vi "OBDservice03.vi"(8 "错误输入（无错误）":errorcluster, 11 "diag ref out输入":T1 {"Diagostic Globals"."Fill Byte" format="%x"; "TesterPresent Message" format="%.0x"; "Selected I/O Mode" items=["CAN", "CAN FD", "CAN FD+BRS", "ECU Determined"]; "DoIP Protocol Version" items=["2010"=1, "2012"=2]; "RX_DL" items=["8"=8, "12"=12, "16"=16, "20"=20, "24"=24, "32"=32, "48"=48, "64"=64]; "TX_DL" items=["8"=8, "12"=12, "16"=16, "20"=20, "24"=24, "32"=32, "48"=48, "64"=64]; "I/O Mode" items=["CAN", "CAN FD", "CAN FD+BRS", "Not yet determined"]}) -> (0 "错误输出":errorcluster, 1 "success?":bool, 2 "dtcs":string[](array[string]), 3 "diag ref out输出":T1 {"Diagostic Globals"."Fill Byte" format="%x"; "TesterPresent Message" format="%.0x"; "Selected I/O Mode" items=["CAN", "CAN FD", "CAN FD+BRS", "ECU Determined"]; "DoIP Protocol Version" items=["2010"=1, "2012"=2]; "RX_DL" items=["8"=8, "12"=12, "16"=16, "20"=20, "24"=24, "32"=32, "48"=48, "64"=64]; "TX_DL" items=["8"=8, "12"=12, "16"=16, "20"=20, "24"=24, "32"=32, "48"=48, "64"=64]; "I/O Mode" items=["CAN", "CAN FD", "CAN FD+BRS", "Not yet determined"]})   [LabVIEW 2018]
uses:
  <vilib>/Automotive Diagnostic Command Set/Diagnostic Transport.llb/Diag Reference.ctl
  <vilib>/Automotive Diagnostic Command Set/Diagnostic Transport.llb/Transport Protocol Selector.ctl
  <vilib>/Automotive Diagnostic Command Set/Diagnostic Transport.llb/DoIP Protocol Version.ctl
  <vilib>/Automotive Diagnostic Command Set/Diagnostic Transport.llb/Diag Globals.ctl
  <vilib>/addons/Automotive Diagnostic Command Set/NI_Automotive Diagnostic Command Set.lvlib
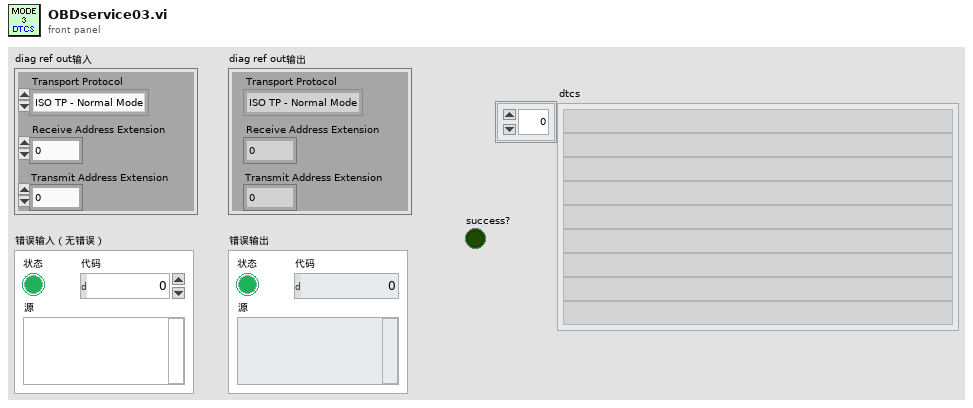
[diagram p1: front panel]
types:
  T1 = typedef "NI_Automotive Diagnostic Command Set.lvlib/Diag Reference.ctl" = cluster{"Diag CAN Handle":u32, "Transport Protocol":T2, "Receive Address Extension":u8, "Transmit Address Extension":u8, "Receive CAN Id":u32, "Transmit CAN Id":u32, "Log Frames ?":bool, "My TP Address":u8, "Other TP Address":u8, "T1":u16, "T2":u16, "T3":u16, "T4":u16, "Tx SN":u8, "Block Size":u8, "Rx SN":u8, "VW TP Initialized?":bool, "Tx block no":u8, "baud rate":u64, "Interface":string, "Channel Diag CAN Handle":u32, "UDP Connection ID":refnum<k16>, "TCP Connection ID":refnum<k5>, "Target IP Addr":u32, "Source Address":u16, "Target Address":u16, "Send Header NACK?":bool, "DLL Handle":u32, "NAD":u8, "Time Stamp read first":dbl, "Time Stamp read last":dbl, "Time Stamp write first":dbl, "Time Stamp write last":dbl, "Time Stamp write":dbl, "Time Stamp read":dbl, " I/O Mode":u32, "FD Baudrate":u64, "TX_DL":u16, "RX_DL":u16, "DoIP Protocol Version":T3, " Selected I/O Mode":u32, "TesterPresent Counter":u32, "TesterPresent Limit":u32, "TesterPresent Tick[ms]":i32, "TesterPresent RequireResponse?":bool, "TesterPresent Stored Ref?":bool, "TesterPresent Message":u8[], "TesterPresent Task Handle":i32, "TesterPresent Semaphore":T4, "Response Plausibility Check":u32, "Default Version?":bool, "Diagostic Globals":T5, "Session-based Properties?":bool}
  T2 = typedef "NI_Automotive Diagnostic Command Set.lvlib/Transport Protocol Selector.ctl" = enum16{"ISO TP - Normal Mode", "ISO TP - Mixed Mode", "VW TP 2.0", "Diagnostics on IP", "ISO TP LIN"}
  T3 = typedef "NI_Automotive Diagnostic Command Set.lvlib/DoIP Protocol Version.ctl" = u8
  T4 = typedef "Semaphore RefNum" = refnum<k1>
  T5 = typedef "NI_Automotive Diagnostic Command Set.lvlib/Diag Globals.ctl" = cluster{"Timeout FC (Bs)":u32, "Timeout CF (Cr)":u32, "Timeout Diag Command":u32, "Receive Block Size (BS)":u8, "Wait Time CF (STmin)":u8, "Max Waits (N_WFTmax)":u8, "Waits to Send (N_WAIT)":i32, "Time between Waits (TW)":u32, "Fill CAN Frames?":bool, "Fill Byte":u32, "Invalid Response as Error?":bool, "Max RspPending Count":u32, "VWTP Command Timeout":u32, "Transport Protocol":T2, "Diag CAN Handle":u32, "DLL Handle":u32, "Timeout RspPending":u32}
  T6 = typedef "Diagnostic Trouble Code.ctl" = cluster{"DTC":u32, "Status":u32, "Add Data":u32}
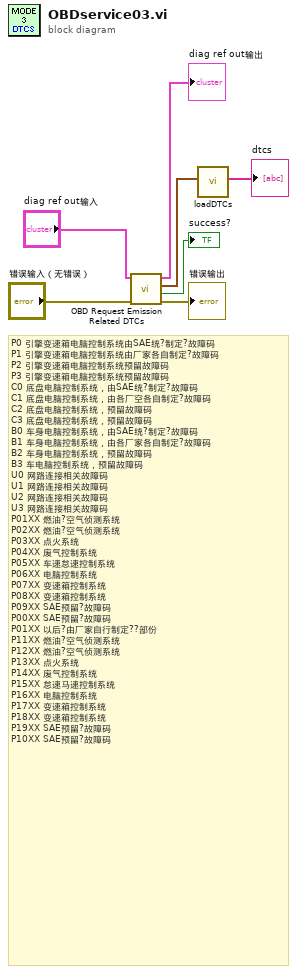
[diagram p0: block diagram]
diagram:
  # "P0 引擎变速箱电脑控制系统由SAE统?制定?故障码\nP1 引擎变速箱电脑控制系统由厂家各自制定?故障码\nP2 引擎变速箱电脑控制系统预留故障码\nP3 引擎变速箱电脑控制系统预留故障码\nC0 底盘电脑控制系统，由SAE统?制定?故障码\nC1 底盘电脑控制系统，由各厂空各自制定?故障码\nC2 底盘电脑控制系统，预留故障码\nC3 底盘电脑控制系统，预留故障码\nB0 车身电脑控制系统，由SAE统?制定?故障码\nB1 车身电脑控制系统，由各厂家各自制定?故障码\nB2 车身电脑控制系统，预留故障码\nB3 车电脑控制系统，预留故障码\nU0 网路连接相关故障码\nU1 网路连接相关故障码\nU2 网路连接相关故障码\nU3 网路连接相关故障码\nP01XX 燃油?空气侦测系统\nP02XX 燃油?空气侦测系统\nP03XX 点火系统\nP04XX 废气控制系统\nP05XX 车速怠速控制系统\nP06XX 电脑控制系统\nP07XX 变速箱控制系统\nP08XX 变速箱控制系统\nP09XX SAE预留?故障码\nP00XX SAE预留?故障码\nP01XX 以后?由厂家自行制定??部份\nP11XX 燃油?空气侦测系统\nP12XX 燃油?空气侦测系统\nP13XX 点火系统\nP14XX 废气控制系统\nP15XX 怠速马速控制系统\nP16XX 电脑控制系统\nP17XX 变速箱控制系统\nP18XX 变速箱控制系统\nP19XX SAE预留?故障码\nP10XX SAE预留?故障码"
  n1 = call <vilib>:"OBD Request Emission Related DTCs.vi"("error in (no error)"="错误输入（无错误）", "diag ref in"="diag ref out输入") -> ("error out"=→"错误输出":errorcluster, "success?"=→"success?":bool, "DTCs"=w2:T6[], "diag ref out"=→"diag ref out输出":T1)  [unwired: 6 in]
  n2 = call "loadDTCs.vi"("DTCs"=w2) -> ("dtcs"=→"dtcs":string[])  [unwired: 10 in]
